vi "Number2Bool.vi"(1 "数值":i32) -> (0 "布尔":bool)   [LabVIEW 2019]
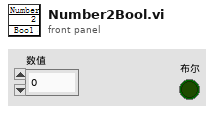
[diagram p1: front panel]
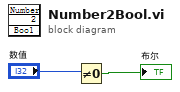
[diagram p0: block diagram]
diagram:
  n1 = Not Equal To 0?(x="数值") -> (x != 0?=→"布尔":bool)
